vi "Main.vi"() -> (2 "DEBUG All Classes":T2[](array[typedef]))   [LabVIEW 2013]
uses:
  Data Structures/JSON/Class.ctl
  Data Structures/JSON/Method.ctl
  Data Structures/JSON/Param.ctl
  Data Structures/JSON/Property.ctl
  <userlib>/ICON Technologies/ICON Maps/lvlib/Map.ctl
  Data Structures/JSON/Simple Struct.ctl
  Data Structures/JSON/TypeConv.ctl
  Param Writers/TypeConv/Action.ctl
  Param Writers/TypeConv/Category.ctl
  <vilib>/addons/JSON API/JSON Value/JSON Value.lvclass
  Param Writers/QObject Writer/QObject Writer.lvclass
  <vilib>/addons/JSON API/JSON Value/Set from JSON string.vi
  <userlib>/ICON Technologies/ICON Maps/lvlib/_Polymorphic Instances/Map_Insert_Variant.vi
  <vilib>/addons/JSON API/Variant JSON/Get as Variant.vi
  <vilib>/addons/JSON API/Get Polymorphic/JSON GetSet.lvlib
  <userlib>/ICON Technologies/ICON Maps/ICON Maps.lvlib
  <vilib>/addons/JSON API/Variant JSON/Variant JSON.lvlib
panel:
  out "Augmented Class Ref Map":T1
  out "Leftover Classes":T1
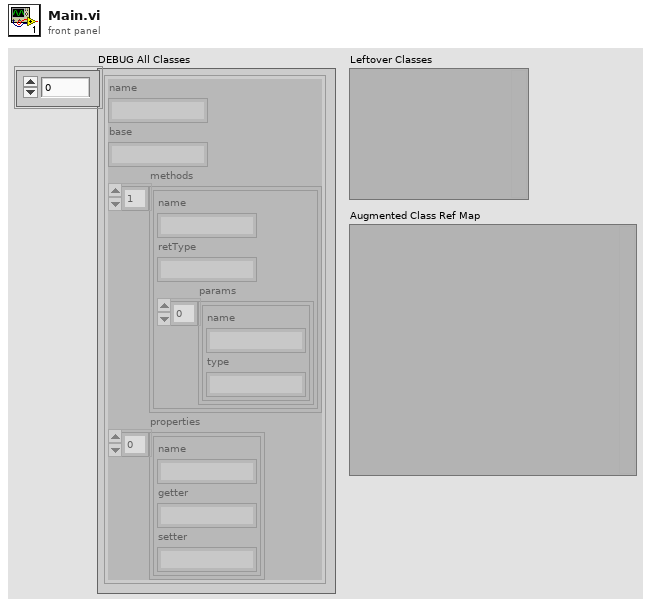
[diagram p1: front panel]
types:
  T1 = typedef "ICON Maps.lvlib/Map.ctl" = variant
  T2 = typedef "Class.ctl" = cluster{"name":string, "base":string, "methods":T3[], "properties":T5[]}
  T3 = typedef "Method.ctl" = cluster{"name":string, "retType":string, "params":T4[]}
  T4 = typedef "Param.ctl" = cluster{"name":string, "type":string}
  T5 = typedef "Property.ctl" = cluster{"name":string, "getter":string, "setter":string}
  T6 = typedef "Category.ctl" = enum16{"Invalid", "Void", "Boolean", "Numeric", "SimpleStruct", "OpaqueStruct", "Identity", "Container"}
  T7 = typedef "Action.ctl" = enum16{"Register Type", "Obtain Writer"}
  T8 = typedef "TypeConv.ctl" = cluster{"name":string, "dllType":string}
  T9 = typedef "Simple Struct.ctl" = cluster{"name":string, "fields":T4[], "methods":T3[]}
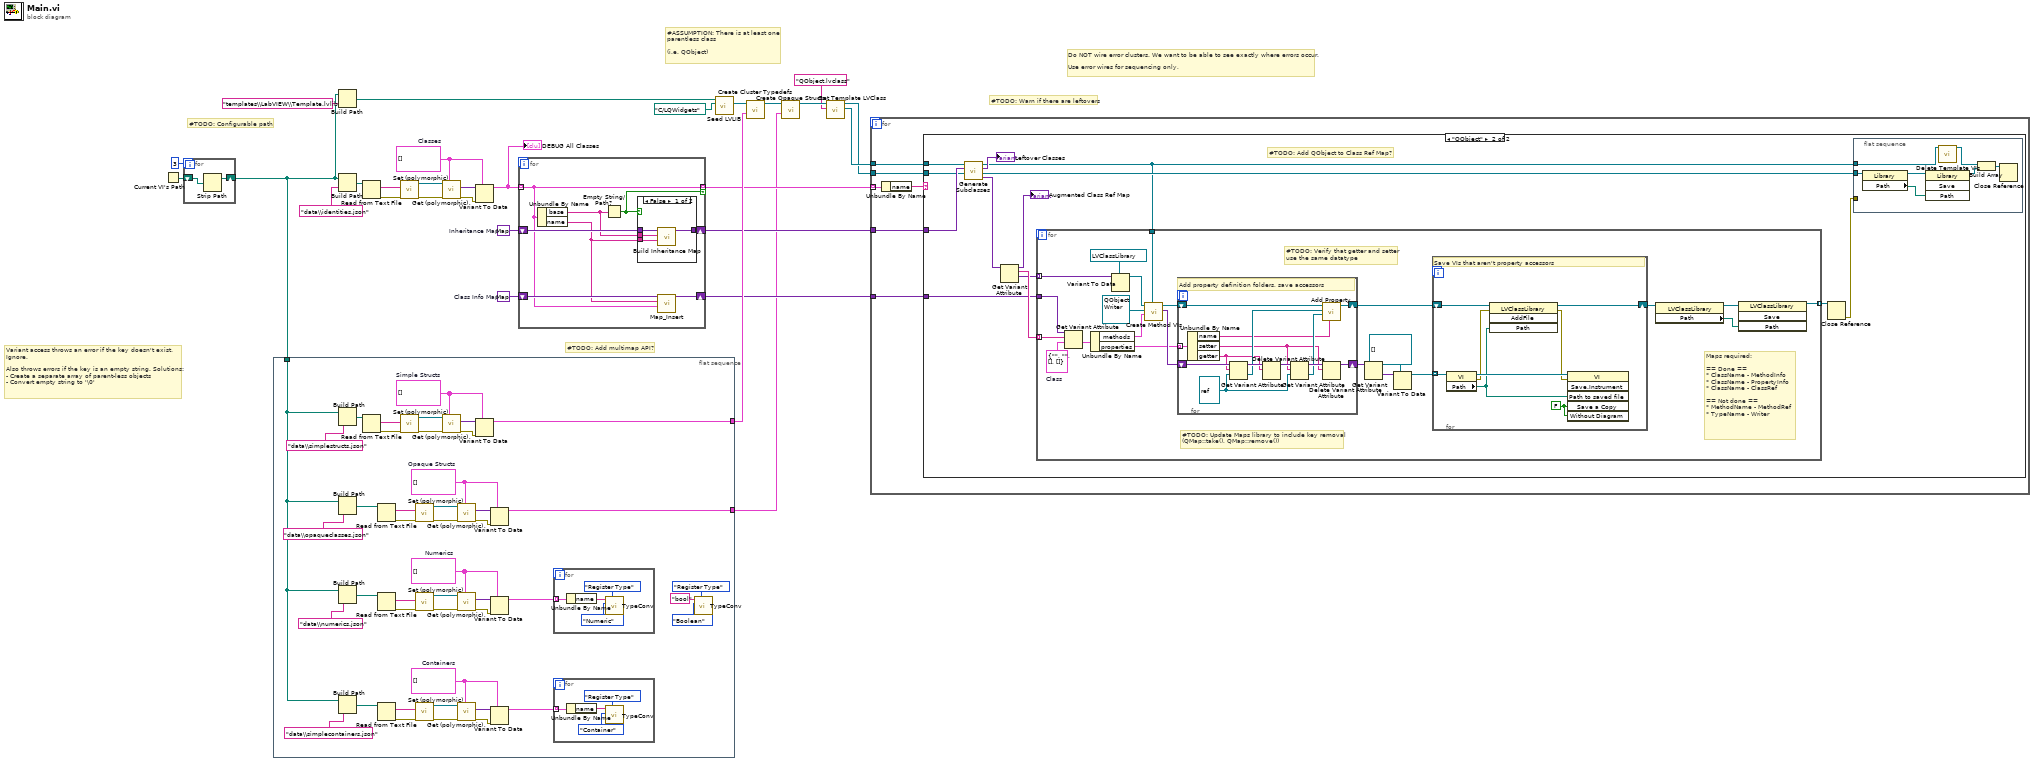
[diagram p0: block diagram]
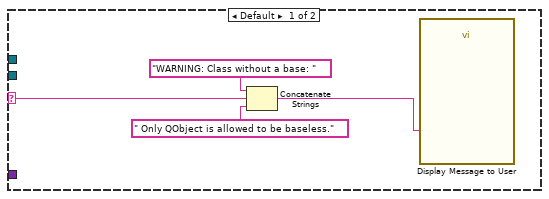
[diagram p2: hidden frame]
diagram:
  w14 = T1 variant  # Class Info Map
  w18 = T1 variant  # Inheritance Map
  w26 = T2[] []  # Classes
  # "#TODO: Add multimap API?"
  # "Do NOT wire error clusters. We want to be able to see exactly where errors occur.\n\nUse error wires for sequencing only,"
  # "#TODO: Warn if there are leftovers"
  # "#ASSUMPTION: There is at least one\nparentless class\n\n(i.e. QObject)"
  # "Variant access throws an error if the key doesn't exist.\nIgnore.\n\nAlso throws errors if the key is an empty string. Solutions:\n- Create a separate array of parent-less objects\n- Convert empty string to '\\0'"
  # "#TODO: Configurable path"
  n1 = Current VI's Path() -> (path=w10:path)
  n2 = for {
    N: 3 -> [_]
    shift-right: [w30] -> w5
    shift-left: w10 -> [w31]
    n3 = Strip Path(path=w31) -> (stripped path=w30:path)  [unwired: 1 out]
  }
  n4 = flat-sequence {
    tunnel: [w75] -> w29
    tunnel: w5 -> [w42]
    tunnel: [w41] -> w4
    frame #0 {
      w37 = T2[] []  # Opaque Structs
      w53 = T8[] []  # Containers
      w59 = T8[] []  # Numerics
      w70 = T9[] []  # Simple Structs
      n5 = Build Path(base path=w42, name or relative path="data\\simplestructs.json") -> (appended path=w74:path)
      n6 = Build Path(base path=w42, name or relative path="data\\opaqueclasses.json") -> (appended path=w40:path)
      n7 = Build Path(base path=w42, name or relative path="data\\numerics.json") -> (appended path=w56:path)
      n8 = Build Path(base path=w42, name or relative path="data\\simplecontainers.json") -> (appended path=w48:path)
      n9 = Read from Text File(file (use dialog)=w74) -> (text=w67:string, error out=w66:errorcluster)  [unwired: 3 in, 2 out]
      n10 = Read from Text File(file (use dialog)=w40) -> (text=w34:string, error out=w33:errorcluster)  [unwired: 3 in, 2 out]
      n11 = Read from Text File(file (use dialog)=w56) -> (text=w62:string, error out=w63:errorcluster)  [unwired: 3 in, 2 out]
      n12 = Read from Text File(file (use dialog)=w48) -> (text=w50:string, error out=w49:errorcluster)  [unwired: 3 in, 2 out]
      n13 = call-poly <vilib>:"Set (polymorphic).vi"("error in (no error)"=w66, "JSON stream"=w67) -> ("error out"=w71:errorcluster, "JSON Value out"=w68:refnum<class "JSON Value.lvclass">)  [unwired: 7 in, 1 out]
      n14 = call-poly <vilib>:"Set (polymorphic).vi"("error in (no error)"=w33, "JSON stream"=w34) -> ("error out"=w38:errorcluster, "JSON Value out"=w35:refnum<class "JSON Value.lvclass">)  [unwired: 7 in, 1 out]
      n15 = call-poly <vilib>:"Set (polymorphic).vi"("error in (no error)"=w63, "JSON stream"=w62) -> ("error out"=w58:errorcluster, "JSON Value out"=w61:refnum<class "JSON Value.lvclass">)  [unwired: 7 in, 1 out]
      n16 = call-poly <vilib>:"Set (polymorphic).vi"("error in (no error)"=w49, "JSON stream"=w50) -> ("error out"=w54:errorcluster, "JSON Value out"=w51:refnum<class "JSON Value.lvclass">)  [unwired: 7 in, 1 out]
      n17 = call-poly <vilib>:"Get (polymorphic).vi"("Variant (Data Type)"=w70, "error in (no error)"=w71, "JSON Scalar in"=w68) -> ("error out"=w72:errorcluster, "Variant out"=w69:variant)  [unwired: 6 in, 1 out]
      n18 = call-poly <vilib>:"Get (polymorphic).vi"("Variant (Data Type)"=w37, "error in (no error)"=w38, "JSON Scalar in"=w35) -> ("error out"=w39:errorcluster, "Variant out"=w36:variant)  [unwired: 6 in, 1 out]
      n19 = call-poly <vilib>:"Get (polymorphic).vi"("Variant (Data Type)"=w59, "error in (no error)"=w58, "JSON Scalar in"=w61) -> ("error out"=w57:errorcluster, "Variant out"=w60:variant)  [unwired: 6 in, 1 out]
      n20 = call-poly <vilib>:"Get (polymorphic).vi"("Variant (Data Type)"=w53, "error in (no error)"=w54, "JSON Scalar in"=w51) -> ("error out"=w55:errorcluster, "Variant out"=w52:variant)  [unwired: 6 in, 1 out]
      n21 = Variant To Data(error in=w72, type=w70, Variant=w69) -> (data=w75:T9[])  [unwired: 1 out]
      n22 = Variant To Data(error in=w39, type=w37, Variant=w36) -> (data=w41:T2[])  [unwired: 1 out]
      n23 = Variant To Data(error in=w57, type=w59, Variant=w60) -> (data=w47:T8[])  [unwired: 1 out]
      n24 = Variant To Data(error in=w55, type=w53, Variant=w52) -> (data=w46:T8[])  [unwired: 1 out]
      n25 = for {
        tunnel: w47 -> [w83] mode=indexing
        n26 = Unbundle By Name(w83) -> ("name"=w82:string)
        n27 = call "TypeConv.vi"("Action"=Action."Register Type", "Category"=Category."Numeric", "Type Name"=w82) -> ()  [unwired: 8 in, 1 out]
      }
      n28 = for {
        tunnel: w46 -> [w79] mode=indexing
        n29 = Unbundle By Name(w79) -> ("name"=w78:string)
        n30 = call "TypeConv.vi"("Action"=Action."Register Type", "Category"=Category."Container", "Type Name"=w78) -> ()  [unwired: 8 in, 1 out]
      }
      n31 = call "TypeConv.vi"("Action"=Action."Register Type", "Category"=Category."Boolean", "Type Name"="bool") -> ()  [unwired: 8 in, 1 out]
    }
  }
  n32 = Build Path(base path=w5, name or relative path="templates\\LabVIEW\\Template.lvlib") -> (appended path=w7:path)
  n33 = Build Path(base path=w5, name or relative path="data\\identities.json") -> (appended path=w24:path)
  n34 = Read from Text File(file (use dialog)=w24) -> (text=w23:string, error out=w22:errorcluster)  [unwired: 3 in, 2 out]
  n35 = call-poly <vilib>:"Set (polymorphic).vi"("error in (no error)"=w22, "JSON stream"=w23) -> ("error out"=w21:errorcluster, "JSON Value out"=w28:refnum<class "JSON Value.lvclass">)  [unwired: 7 in, 1 out]
  n36 = call-poly <vilib>:"Get (polymorphic).vi"("Variant (Data Type)"=w26, "error in (no error)"=w21, "JSON Scalar in"=w28) -> ("error out"=w20:errorcluster, "Variant out"=w27:variant)  [unwired: 6 in, 1 out]
  n37 = Variant To Data(error in=w20, type=w26, Variant=w27) -> (data=w19:T2[])  [unwired: 1 out]
  "DEBUG All Classes" <- w19
  n38 = for {
    tunnel: w19 -> [w86] mode=indexing
    shift-right: [w91] -> w15
    shift-left: w18 -> [w90]
    tunnel: [w86] -> w17 mode=indexing if=w88
    shift-right: [w85] -> w13
    shift-left: w14 -> [w87]
    n39 = Unbundle By Name(w86) -> ("base"=w89:string, "name"=w84:string)
    n40 = Empty String/Path?(string/path=w89) -> (empty?=w88:bool)
    n41 = case shown="False" w88 {
      tunnel: [w95 w96] -> w91
      tunnel: w84 -> [w94 _]
      tunnel: w90 -> [w93 w96]
      tunnel: w89 -> [w92 _]
      frame False {
        n42 = call "Build Inheritance Map.vi"("Subclass Name"=w94, "Base Class Name"=w92, "Inheritance Map"=w93) -> ("Augmented Inheritance Map"=w95:T1)  [unwired: 8 in]
      }
      frame True {
      }
    }
    n43 = call-poly <userlib>:"Map_Insert.vi"("Value"=w86, "Key"=w84, "Map In"=w87) -> ("Map Out"=w85:T1)  [unwired: 8 in]
  }
  n44 = call "Seed LVLIB.vi"("Output Dir"=path "C:/LQWidgets", "LVLib Template Path"=w7) -> ("New LVLib"=w6:refnum<vi>)  [unwired: 9 in]
  n45 = call "Create Cluster Typedefs.vi"("Simple Structs"=w29, "LVLib"=w6) -> ("LVLib Dup"=w3:refnum<vi>)  [unwired: 9 in]
  n46 = call "Create Opaque Structs.vi"("Opaque Structs"=w4, "LVLib"=w3) -> ("LVLib Dup"=w2:refnum<vi>)  [unwired: 9 in]
  n47 = call "Get Template LVClass.vi"("LVClass Simple Name"="QObject.lvclass", "LVLib"=w2) -> ("Object Ref"=w16:refnum<vi>, "LVLib Dup"=w11:refnum<vi>)  [unwired: 8 in]
  n48 = for {
    tunnel: w17 -> [w102] mode=indexing
    tunnel: w16 -> [w100]
    tunnel: w15 -> [w99]
    tunnel: w13 -> [w98]
    tunnel: w11 -> [w97]
    n49 = Unbundle By Name(w102) -> ("name"=w101:string)
    n50 = case shown="\"QObject\"" w101 {
      selector: w101 -> [w105 _]
      tunnel: w99 -> [_ w118]
      tunnel: w100 -> [_ w119]
      tunnel: w98 -> [_ w113]
      tunnel: w97 -> [_ w111]
      frame Default {
        n51 = Concatenate Strings("WARNING: Class without a base: " ("string"), w105, " Only QObject is allowed to be baseless." ("string")) -> (w103:string)
        n52 = call "Display Message to User"("Message"=w103) -> ()  [unwired: 9 in, 2 out]
      }
      frame "QObject" {
        # "#TODO: Add QObject to Class Ref Map?"
        n53 = call "Generate Subclasses.vi"("Owning LVLib"=w111, "Inheritance Map"=w118, "Base Class"=w119) -> ("Augmented Class Ref Map"=w110:T1, "Owning LVLib Dup"=w117:refnum<vi>, "Reduced Inheritance Map"=→"Leftover Classes":T1, "Base Class Dup"=w107:refnum<vi>)  [unwired: 5 in]
        n54 = Get Variant Attribute(Variant=w110) -> (duplicate Variant=→"Augmented Class Ref Map":variant, names=w115:string[], values=w114:variant[])  [unwired: 3 in, 1 out]
        n55 = for {
          tunnel: w115 -> [w144] mode=indexing
          tunnel: w114 -> [w148] mode=indexing
          tunnel: w113 -> [w145]
          tunnel: [w129] -> w112 mode=indexing
          tunnel: w107 -> [w128]
          w143 = T2 {"name"="", "base"="", "methods"=[], "properties"=[]}  # Class
          # "#TODO: Verify that getter and setter\nuse the same datatype"
          # "#TODO: Update Maps library to include key removal\n(QMap::take(), QMap::remove())"
          # "Maps required:\n\n== Done ==\n* ClassName - MethodInfo\n* ClassName - PropertyInfo\n* ClassName - ClassRef\n\n== Not done ==\n* MethodName - MethodRef\n* TypeName - Writer"
          n56 = Get Variant Attribute(Variant=w145, name=w144, default value (empty Variant)=w143) -> (value=w142:T2)  [unwired: 1 in, 3 out]
          n57 = Unbundle By Name(w142) -> ("methods"=w141:T3[], "properties"=w134:T5[])
          n58 = Variant To Data(type=refnum<vi> refnum ("QObject"), Variant=w148) -> (data=w146:refnum<vi>)  [unwired: 1 in, 1 out]
          n59 = call "Create Method VIs.vi"("Template Class"=w128, "Methods"=w141, "Class Param Writer"=refnum<class "QObject Writer.lvclass"> refnum ("QObject Writer.lvclass"), "Class"=w146) -> ("Method Ref Map"=w135:T1, "Class Dup"=w136:refnum<vi>)  [unwired: 6 in]
          n60 = for {
            shift-right: [w169] -> w137
            shift-left: w136 -> [w170]
            shift-right: [w162] -> w140
            shift-left: w135 -> [w168]
            tunnel: w134 -> [w160] mode=indexing
            w161 = refnum<vi> refnum ("reference out")
            # "Add property definition folders, save accessors"
            n61 = Unbundle By Name(w160) -> ("name"=w159:string, "setter"=w158:string, "getter"=w157:string)
            n62 = Get Variant Attribute(Variant=w168, name=w157, default value (empty Variant)=w161) -> (duplicate Variant=w167:variant, value=w166:refnum<vi>)  [unwired: 1 in, 2 out]
            n63 = Delete Variant Attribute(6:w157, 7:w167) -> (3:w164:variant)  [unwired: 1 in, 2 out]
            n64 = Get Variant Attribute(Variant=w164, name=w158, default value (empty Variant)=w161) -> (duplicate Variant=w165:variant, value=w163:refnum<vi>)  [unwired: 1 in, 2 out]
            n65 = call "Add Property.vi"("Property Name"=w159, "Setter"=w163, "Getter"=w166, "Class"=w170) -> ("Class Dup"=w169:refnum<vi>)  [unwired: 7 in]
            n66 = Delete Variant Attribute(6:w158, 7:w165) -> (3:w162:variant)  [unwired: 1 in, 2 out]
          }
          n67 = Get Variant Attribute(Variant=w140) -> (values=w139:variant[])  [unwired: 3 in, 3 out]
          n68 = Variant To Data(type=refnum<vi>[] [], Variant=w139) -> (data=w130:refnum<vi>[])  [unwired: 1 in, 1 out]
          n69 = for {
            tunnel: w130 -> [w154] mode=indexing
            shift-right: [w151] -> w133
            shift-left: w137 -> [w153]
            w155 = FALSE ("Save a Copy")
            # "Save VIs that aren't property accessors"
            n70 = property class="VI"(reference=w154) -> (reference out=w156:refnum<vi>, error out=w149:errorcluster, "Path"=w152:path)  [unwired: 1 in]
            n71 = invoke class="LVClassLibrary" method="AddFile"(reference=w153, error in=w149, "Path"=w152) -> (reference out=w151:refnum<vi>, error out=w150:errorcluster)  [unwired: 1 in, 2 out]
            n72 = invoke class="VI" method="Save.Instrument"(reference=w156, error in=w150, "Path to saved file"=w152, "Save a Copy"=w155, "Without Diagram"=w155) -> ()  [unwired: 1 in, 6 out]
          }
          n73 = property class="LVClassLibrary"(reference=w133) -> (reference out=w132:refnum<vi>, "Path"=w131:path)  [unwired: 1 in, 1 out]
          n74 = invoke class="LVClassLibrary" method="Save"(reference=w132, "Path"=w131) -> (reference out=w129:refnum<vi>)  [unwired: 2 in, 3 out]
        }
        n75 = Close Reference(reference=w112) -> (error out=w108:errorcluster)  [unwired: 1 in]
        n76 = flat-sequence {
          tunnel: w117 -> [w126]
          tunnel: w108 -> [_]
          tunnel: w107 -> [w121]
          frame #0 {
            n77 = property class="Library"(reference=w126) -> (reference out=w125:refnum<vi>, "Path"=w124:path)  [unwired: 1 in, 1 out]
            n78 = invoke class="Library" method="Save"(reference=w125, "Path"=w124) -> (reference out=w123:refnum<vi>)  [unwired: 2 in, 3 out]
            n79 = call "Delete Template VIs.vi"("LVClass"=w121) -> ("LVClass Dup"=w120:refnum<vi>)  [unwired: 10 in]
            n80 = Build Array(w120, w123) -> (w122:refnum<vi>[])
            n81 = Close Reference(reference=w122) -> ()  [unwired: 1 in, 1 out]
          }
        }
      }
    }
  }
